vi "Set Frame Type.vi"(8 "error in (no error)":errorcluster caption="entrée d'erreur (pas d'erreur)", 10 "Frame Type":enum16{"Teach IN", "Normal Mode"}(ring), 11 "Wait_Frame_ERP1 en entrée":refnum<class "Wait_Frame_ERP1.lvclass">) -> (0 "error out":errorcluster caption="sortie d'erreur", 3 "Wait_Frame_ERP1 en sortie":refnum<class "Wait_Frame_ERP1.lvclass">)   [LabVIEW 2020, in "Library Test.lvlib" / "Wait_Frame_ERP1.lvclass"]
uses:
  Wait_Frame_ERP1.lvclass
  Wait_Frame_ERP1.lvclass/Wait_Frame_ERP1.ctl
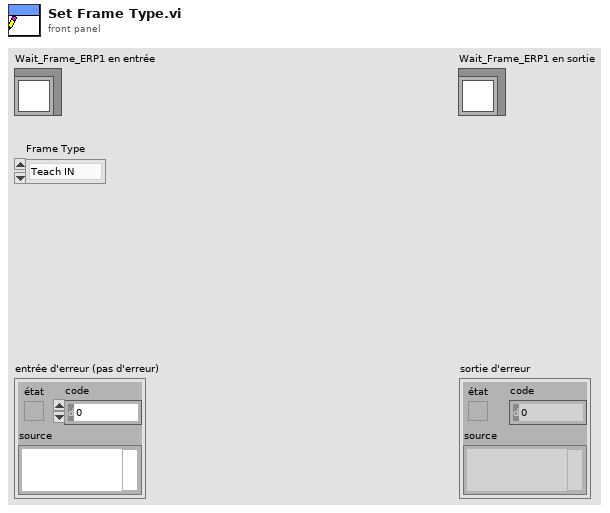
[diagram p1: front panel]
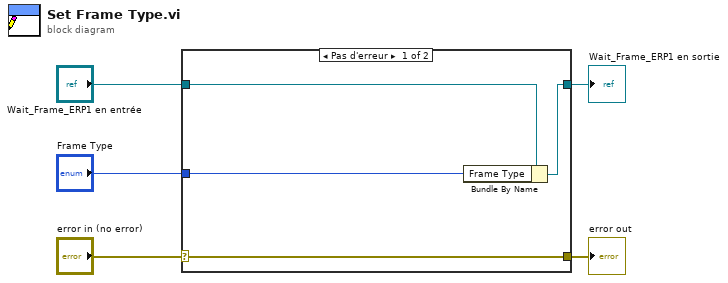
[diagram p0: block diagram]
diagram:
  n1 = case shown="Pas d'erreur" "error in (no error)" {
    selector: "error in (no error)" -> [w9 w10]
    tunnel: [w9 w10] -> w4
    tunnel: [w7 w11] -> w2
    tunnel: "Wait_Frame_ERP1 en entrée" -> [w8 w11]
    tunnel: "Frame Type" -> [w6 _]
    frame No Error {
      n2 = Bundle By Name(cluster=w8, "Frame Type"=w6) -> (w7:refnum<class "Wait_Frame_ERP1.lvclass">)
    }
    frame Error {
    }
  }
  "error out" <- w4
  "Wait_Frame_ERP1 en sortie" <- w2
